vi "Read Power Actual (Single).vi"(8 "error in":errorcluster, 9 "Channel Index":i32=1, 11 "Cycler in":refnum<class "Cycler.lvclass">) -> (0 "error out":errorcluster, 1 "Changed or First Call?":bool, 2 "Power":dbl, 3 "Cycler out":refnum<class "Cycler.lvclass">)   [LabVIEW 2023, in "Cycler.lvclass"]
uses:
  Cycler.lvclass
  Cycler.lvclass/Cycler.ctl
  <vilib>/ADAS Replay HIL/Channels/Tag Wrapper/Tag Wrapper.lvlib
  <vilib>/ADAS Replay HIL/Channels/Tag Wrapper/Polymorphic/Read Channel (Double).vi
  77db10b4-460d-4622-b970-a092dfc26952.vi
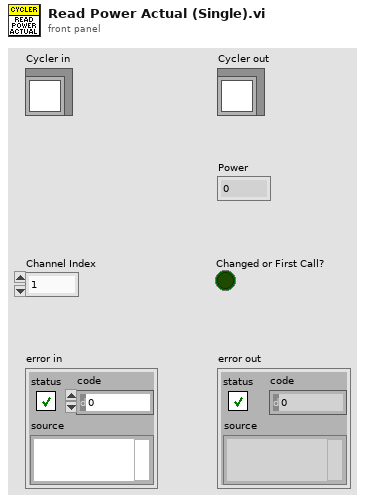
[diagram p1: front panel]
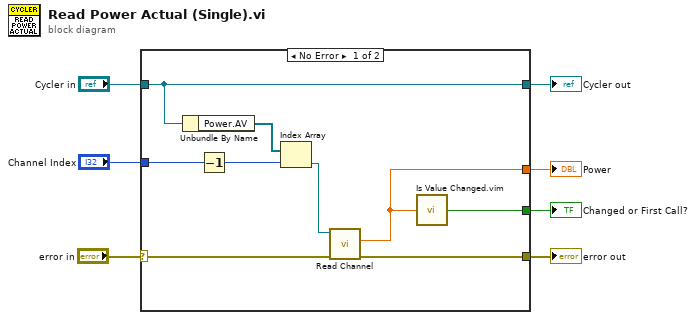
[diagram p0: block diagram]
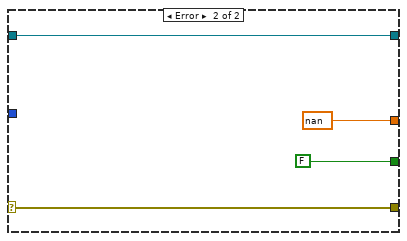
[diagram p2: hidden frame]
diagram:
  n1 = case shown="No Error" "error in" {
    selector: "error in" -> [w15 w19]
    tunnel: [w14 w19] -> w6
    tunnel: [w16 w20] -> w4
    tunnel: "Cycler in" -> [w16 w20]
    tunnel: [w9 nan ("Value out")] -> w3
    tunnel: "Channel Index" -> [w11 _]
    tunnel: [w8 FALSE ("changed or first call?")] -> w1
    frame No Error {
      n2 = Unbundle By Name(w16) -> ("Power.AV"=w13:refnum<k21>[])
      n3 = Decrement(x=w11) -> (x-1=w10:i32)
      n4 = Index Array(array=w13, index=w10) -> (element=w12:refnum<k21>)
      n5 = call-poly <vilib>:"Read Channel.vi"("error in"=w15, "ADAS HIL Channel in"=w12) -> ("error out"=w14:errorcluster, "Value out"=w9:dbl)  [unwired: 6 in, 2 out]
      n6 = call "Is Value Changed.vim"("value"=w9) -> ("changed or first call?"=w8:bool)
    }
    frame Error {
    }
  }
  "error out" <- w6
  "Cycler out" <- w4
  "Power" <- w3
  "Changed or First Call?" <- w1
